vi "testRunViWithInput.vi"(8 "error in (no error)":errorcluster) -> (0 "error out":errorcluster)   [LabVIEW 2018]
uses:
  src/SalProcess/SalProcess.lvclass
  src/VariantTool/getValFromVariant_enum.vi
  <vilib>/addons/_JKI Toolkits/Caraya/classes/Assert/Assert Equal Value_Variant.vi
  src/VariantTool/getValFromVariant_double.vi
  <vilib>/addons/_JKI Toolkits/Caraya/classes/Test/Test.lvclass
  <vilib>/addons/_JKI Toolkits/Caraya/classes/Assert/Assert.lvclass
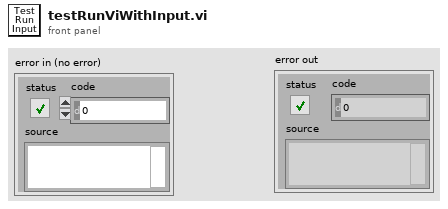
[diagram p1: front panel]
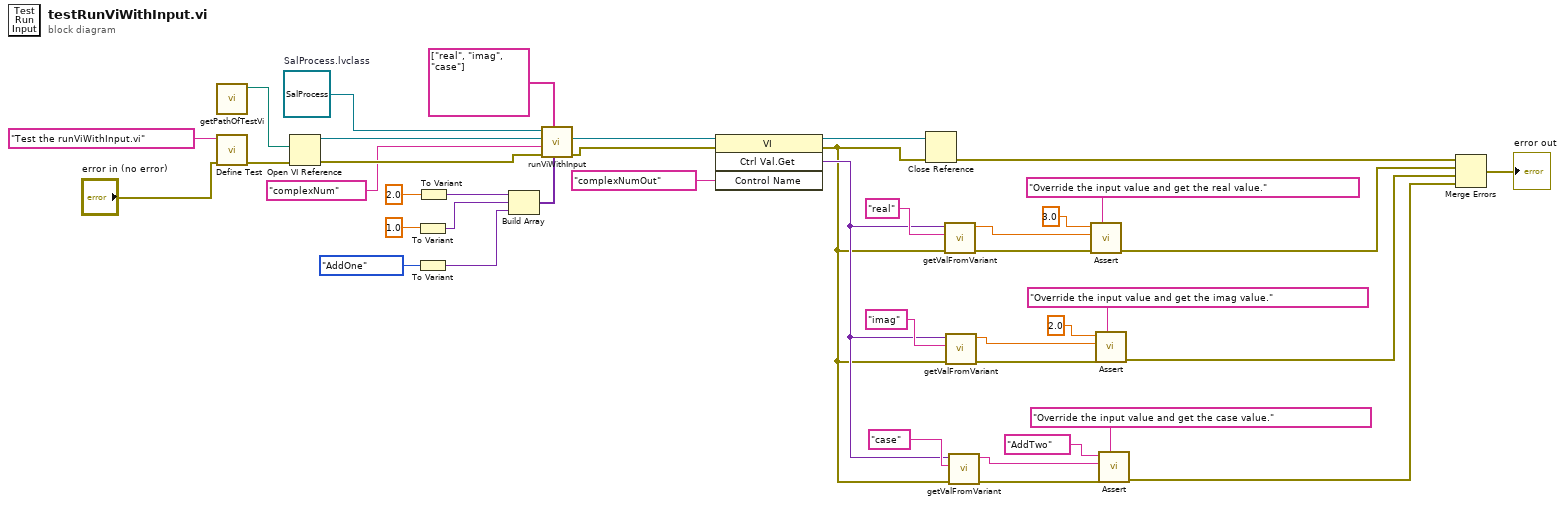
[diagram p0: block diagram]
diagram:
  w39 = refnum<class "SalProcess.lvclass"> refnum  # SalProcess.lvclass
  n1 = call "getPathOfTestVi.vi"() -> ("pathOfTestVi"=w25:path)  [unwired: 11 in]
  n2 = call <vilib>:"Define Test.vi"("error in (no error)"="error in (no error)", "Label (VI Title)"="Test the runViWithInput.vi") -> ("error out"=w40:errorcluster)  [unwired: 9 in]
  n3 = Open VI Reference(vi path=w25, error in (no error)=w40) -> (vi reference=w37:refnum<vi>, error out=w38:errorcluster)  [unwired: 4 in]
  n4 = To Variant(anything=1.0) -> (Variant=w31:variant)
  n5 = To Variant(anything=enum16{"", "AddOne", "AddTwo"}."AddOne" ("case")) -> (Variant=w10:variant)
  n6 = To Variant(anything=2.0) -> (Variant=w32:variant)
  n7 = Build Array(w32, w31, w10) -> (w30:variant[])
  n8 = call "runViWithInput.vi"("valueElement"=w30, "nameElement"=string[] ["real", "imag", "case"], "error in (no error)"=w38, "clusterNameInput"="complexNum", "referenceIn"=w37, "SalProcess in"=w39) -> ("error out"=w27:errorcluster, "referenceOut"=w28:refnum<vi>)  [unwired: 3 in, 1 out]
  n9 = invoke on="Invoke Node" class="VI" method="Ctrl Val.Get"(reference=w28, error in=w27, "Control Name"="complexNumOut") -> (reference out=w26:refnum<vi>, error out=w3:errorcluster, "Get Control Value Variant"=w4:variant)  [unwired: 1 in, 1 out]
  n10 = Close Reference(reference=w26, error in (no error)=w3) -> (error out=w14:errorcluster)
  n11 = call-poly "getValFromVariant.vi"("error in (no error)"=w3, "name"="real", "variant"=w4) -> ("error out"=w22:errorcluster, "value"=w15:dbl)  [unwired: 7 in]
  n12 = call-poly "getValFromVariant.vi"("error in (no error)"=w3, "name"="imag", "variant"=w4) -> ("error out"=w17:errorcluster, "value"=w16:dbl)  [unwired: 7 in]
  n13 = call-poly "getValFromVariant.vi"("error in (no error)"=w3, "name"="case", "variant"=w4) -> ("error out"=w6:errorcluster, "value"=w5:string)  [unwired: 7 in]
  n14 = call-poly <vilib>:"Assert.vi"("Label"="Override the input value and get the real value.", "error in (no error)"=w22, "Y"=w15, "X"=3.0) -> ("error out"=w13:errorcluster)  [unwired: 7 in]
  n15 = call-poly <vilib>:"Assert.vi"("Label"="Override the input value and get the imag value.", "error in (no error)"=w17, "Y"=w16, "X"=2.0) -> ("error out"=w12:errorcluster)  [unwired: 7 in]
  n16 = call-poly <vilib>:"Assert.vi"("Label"="Override the input value and get the case value.", "error in (no error)"=w6, "Y"=w5, "X"="AddTwo") -> ("error out"=w2:errorcluster)  [unwired: 7 in]
  n17 = Merge Errors(w14, w13, w12, w2) -> (→"error out":errorcluster)
